vi "AngleToShoulderEncoder.vi"(11 "angle(deg)":dbl) -> (3 "encoderPulses":i32)   [LabVIEW 2018]
uses:
  Arm Constants.vi
panel:
  in  "Boolean":bool
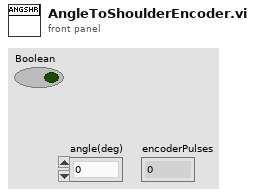
[diagram p1: front panel]
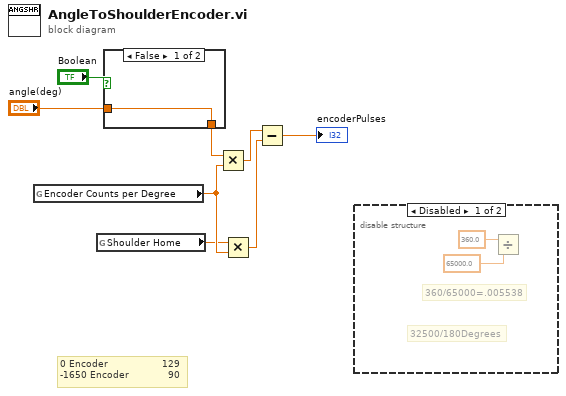
[diagram p0: block diagram]
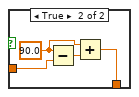
[diagram p2: hidden frame]
diagram:
  # "0 Encoder                  129\n-1650 Encoder             90"
  n1 = global read "Arm Constants.vi" "Encoder Counts per Degree"() -> (w8:dbl)
  n2 = global read "Arm Constants.vi" "Shoulder Home"() -> (w5:dbl)
  n3 = case shown="False" "Boolean" {
    tunnel: "angle(deg)" -> [w9 w11]
    tunnel: [w9 w10] -> w2
    frame False {
    }
    frame True {
      w12 = 90.0 ("x")
      n4 = Subtract(x=w12, y=w11) -> (x-y=w13:dbl)
      n5 = Add(x=w12, y=w13) -> (x+y=w10:dbl)
    }
  }
  n6 = Multiply(x=w2, y=w8) -> (x*y=w6:dbl)
  n7 = Multiply(x=w5, y=w8) -> (x*y=w7:dbl)
  n8 = Subtract(x=w6, y=w7) -> (x-y=→"encoderPulses":dbl)
  n9 = disable-structure shown="Disabled" {
    frame Disabled {
      # "360/65000=.005538"
      # "32500/180Degrees"
      n10 = Divide(x=360.0, y=65000.0) -> ()  [unwired: 1 out]
    }
    frame Enabled {
    }
  }
